vi "HEWH Get Statistics.vi"(4 "Flow Selector":T1, 6 "Emerson Flow Meter Data Output":T2, 8 "Error In":errorcluster, 10 "Elapsed Time (sec)":dbl, 11 "Core HEWH Data in":T3 {"Test Patten Setup"."PRAT/RLT Sequence"."Time" format="%<%H:%M:%S>t"; "Test Patten Setup"."Total Gallons Schedule" format="%.2f"}) -> (0 "Error Out":errorcluster, 1 "Mean,SD,Var,Max,Min Array":string[][](array[string]), 3 "Draw Stats Out":dbl[][](array[numeric]))   [LabVIEW 2016]
uses:
  Type Definitions/HEWH Output Information.ctl
  Type Definitions/HEWH Draw Pattern Setup.ctl
  Type Definitions/PRAT Test.ctl
  Utility/Save File/File Setup (Public)/Type Definition/Save File HEWH Heating Control Mode.ctl
  Draw Water Specific/Type Definitions/Terminate Draw Conditions.ctl
  Type Definitions/HEWH Start Conditions.ctl
  Draw Water Specific/Type Definitions/Check Special Condtions.ctl
  Draw Water Specific/Type Definitions/HEWH Special Condition Check.ctl
  Type Definitions/HEWH Draw Flag ENUM.ctl
  Type Definitions/HEWH Specific DAQ.ctl
  Type Definitions/HEWH Power Data.ctl
  Type Definitions/HEWH Power Elements.ctl
  Utility/Type Definitions/UTILITY Power Analyzer.ctl
  Type Definitions/HEWH Calc and Calibration.ctl
  Utility/Save File/File Setup (Public)/Type Definition/Save File DOE LabView Program.ctl
  Custom Instrument Control/MW100/Type Definitions/Station ID Selector.ctl
  Range/Type Definitions/RANGE ANSI Rate.ctl
  Drivers/Emerson 5700 Transmitter/Type Definitions/Emerson 5700 Data.ctl
  Type Definitions/Flow Meter Selector.ctl
  Utility/Save File/File Setup.lvlib
panel:
  # "Draw Pattern Setup (24 Hour)"
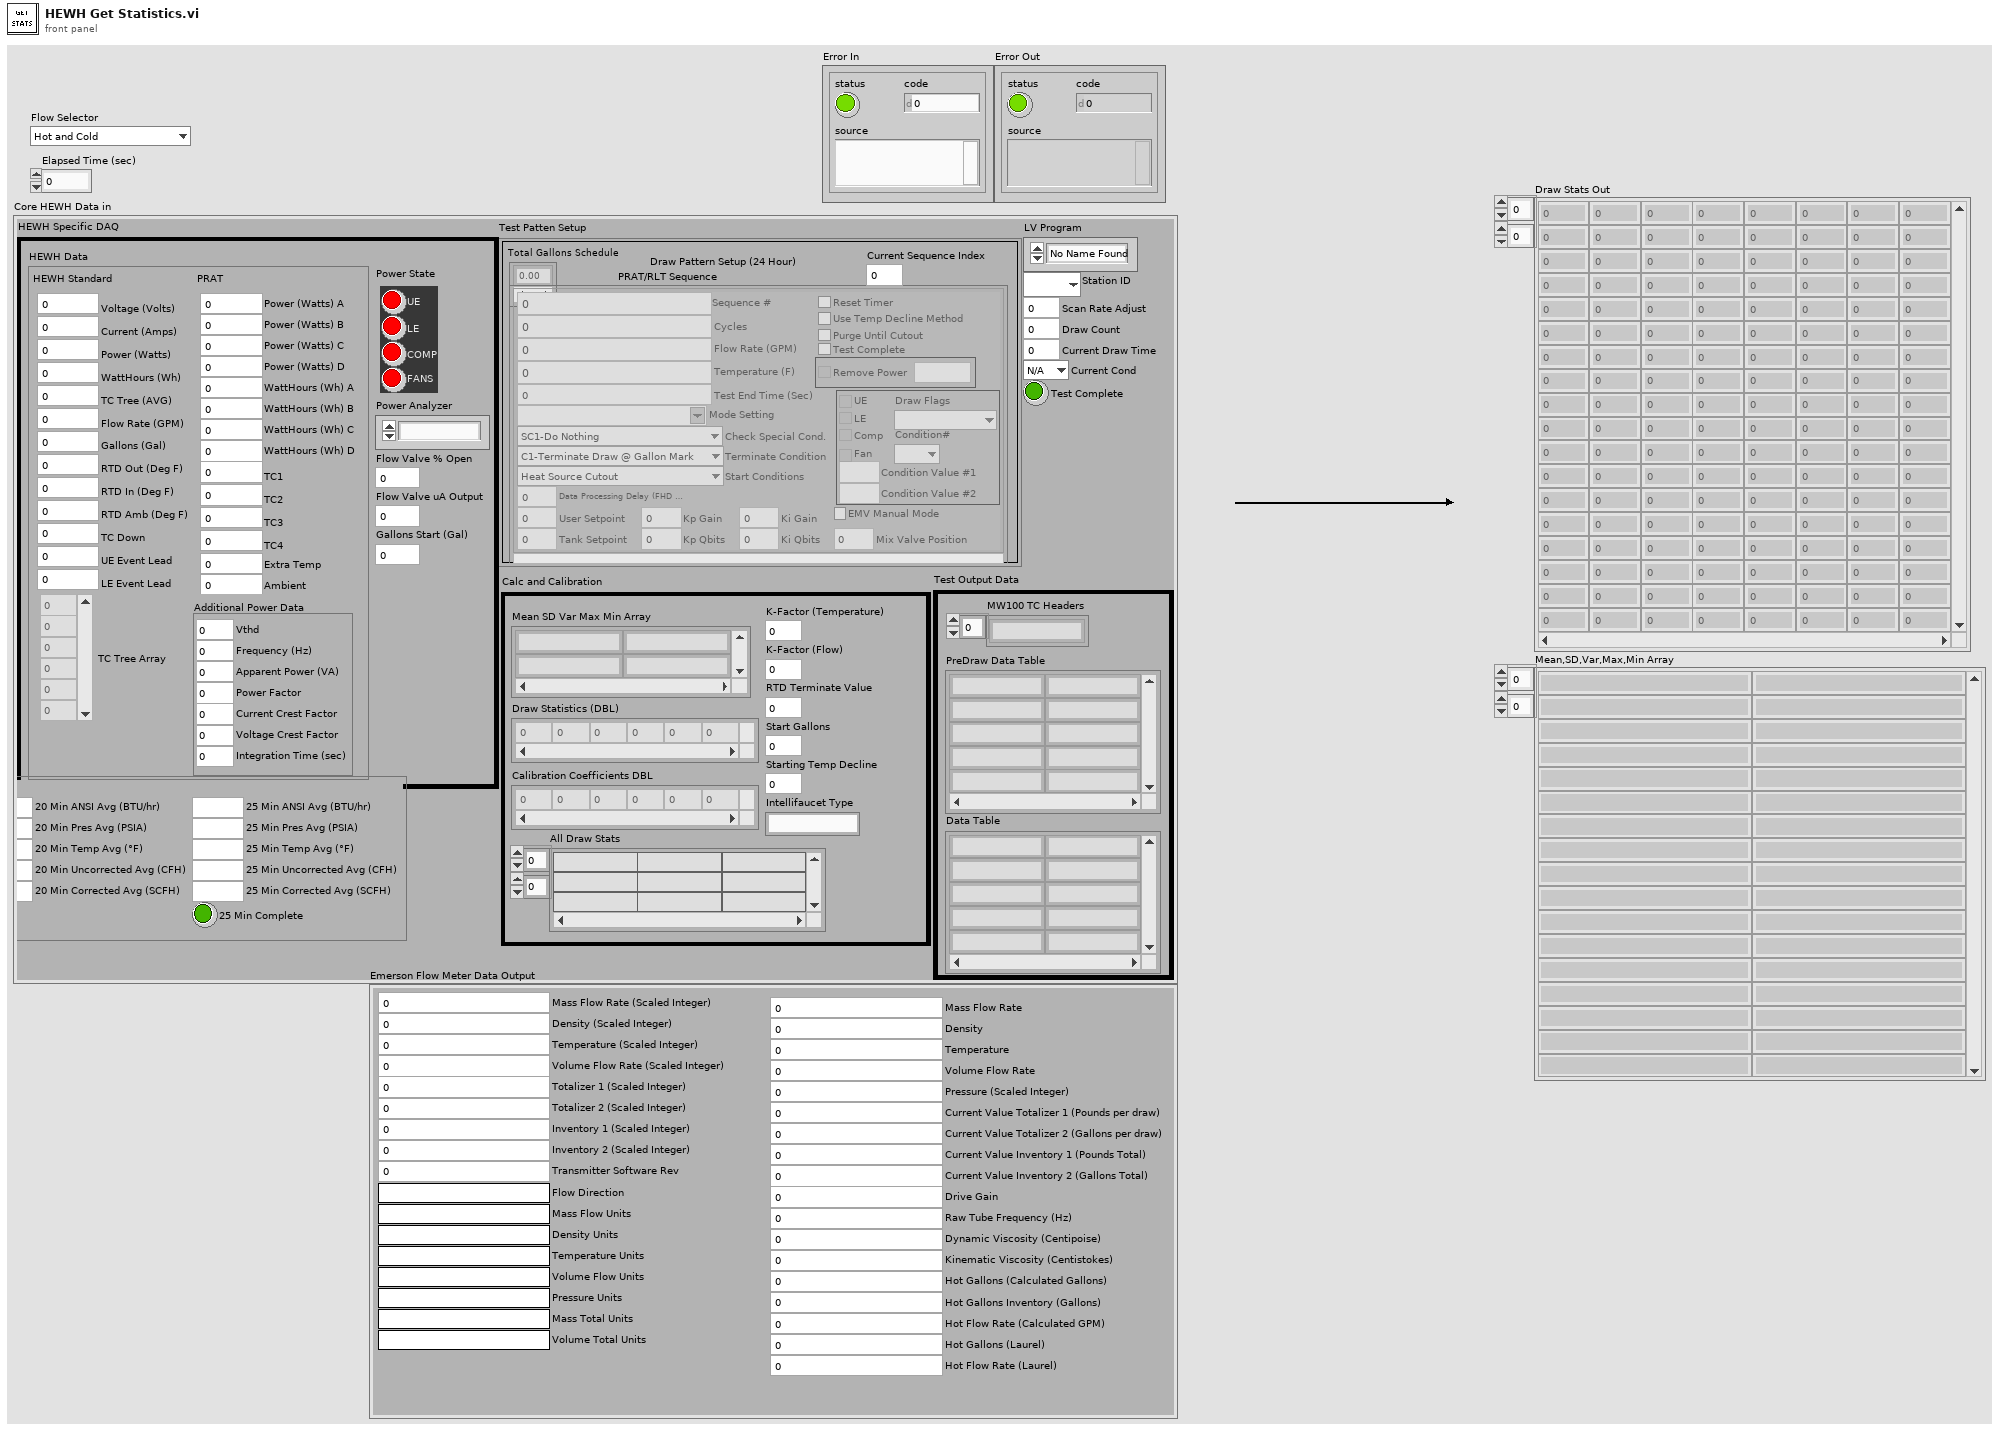
[diagram p1: front panel]
types:
  T1 = typedef "Flow Meter Selector.ctl" = enum16{"Hot and Cold", "Hot", "Cold", "None"}
  T2 = typedef "Emerson 5700 Data.ctl" = cluster{"Mass Flow Rate (Scaled Integer)":u16, "Density (Scaled Integer)":u16, "Temperature (Scaled Integer)":u16, "Volume Flow Rate (Scaled Integer)":u16, "Totalizer 1 (Scaled Integer)":u16, "Totalizer 2 (Scaled Integer)":u16, "Transmitter Software Rev":u16, "Flow Direction":string, "Mass Flow Units":string, "Density Units":string, "Temperature Units":string, "Volume Flow Units":string, "Pressure Units":string, "Mass Total Units":string, "Volume Total Units":string, "Inventory 1 (Scaled Integer)":u16, "Inventory 2 (Scaled Integer)":u16, "Mass Flow Rate":dbl, "Density":dbl, "Temperature":dbl, "Volume Flow Rate":dbl, "Pressure (Scaled Integer)":u16, "Current Value Totalizer 1 (Pounds per draw)":dbl, "Current Value Totalizer 2 (Gallons per draw)":dbl, "Current Value Inventory 1 (Pounds Total)":dbl, "Current Value Inventory 2 (Gallons Total)":dbl, "Drive Gain":dbl, "Raw Tube Frequency (Hz)":dbl, "Dynamic Viscosity (Centipoise)":dbl, "Kinematic Viscosity (Centistokes)":dbl, "Hot Gallons (Calculated Gallons)":dbl, "Hot Flow Rate (Calculated GPM)":dbl, "Hot Gallons Inventory (Gallons)":dbl, "Hot Flow Rate (Laurel)":dbl, "Hot Gallons (Laurel)":dbl}
  T3 = typedef "HEWH Output Information.ctl" = cluster{"Scan Rate Adjust":dbl, "Draw Count":i32, "Test Patten Setup":T4, "HEWH Specific DAQ":T12, "Test Output Data":cluster{"PreDraw Data Table":string[][], "Data Table":string[][], "MW100 TC Headers":string[]}, "Calc and Calibration":T16, "Current Draw Time":dbl, "LV Program":T17, "Station ID":T18, "Current Cond":T10, "Test Complete":bool, "ANSI Rate":T19}
  T4 = typedef "HEWH Draw Pattern Setup.ctl" = cluster{"Total Gallons Schedule":dbl[], "PRAT/RLT Sequence":T5[], "Current Sequence Index":i32}
  T5 = typedef "PRAT Test.ctl" = cluster{"Sequence #":dbl, "Cycles":i32, "Mode Setting":T6, "Flow Rate (GPM)":dbl, "Temperature (F)":dbl, "Reset Timer":bool, "Use Temp Decline Method":bool, "Terminate Condition":T7, "Condition Value #1":dbl, "UE":bool, "LE":bool, "Comp":bool, "Fan":bool, "Test End Time (Sec)":dbl, "Purge Until Cutout":bool, "Start Conditions":T8, "Condition Value #2":dbl, "Remove Power":bool, "Time":dbl, "Check Special Cond.":T9, "Condition#":T10, "Draw Flags":T11, "Data Processing Delay (FHD 15sec, UEF 5 Sec)":dbl, "Test Complete":bool, "User Setpoint":dbl, "Tank Setpoint":dbl, "Kp Gain":dbl, "Kp Qbits":dbl, "Ki Gain":dbl, "Ki Qbits":dbl, "Mix Valve Position":i16, "EMV Manual Mode":bool}
  T6 = typedef "File Setup.lvlib/Save File HEWH Heating Control Mode.ctl" = string
  T7 = typedef "Terminate Draw Conditions.ctl" = enum16{"C1-Terminate Draw @ Gallon Mark", "C2-Special Last Draw (HU Test)", "C3-RTD Out <=", "C4-Mean Tank Temp <=", "C5-Decrease RTD Out (Deg F)", "C6-Time (Seconds)", "C7-Until Any Heat Source", "C8-Specific Heat Source", "C9-Do Nothing"}
  T8 = typedef "HEWH Start Conditions.ctl" = enum16{"Heat Source Cutout", "At Time (Seconds)", "Every X (Seconds)", "T2 >= X° Below Setpoint", "Seconds From Complete", "Wait for LE & Comp Cutout", "Wait for Comp Cutout", "Wait for LE Cutout", "Wait for UE Cutout"}
  T9 = typedef "Check Special Condtions.ctl" = enum16{"SC1-Do Nothing", "SC2-Check Heat Source (On-C2/Off-C1)", "SC3-Check Skip Condition", "SC4-Check Heat Source ON/Fail"}
  T10 = typedef "HEWH Special Condition Check.ctl" = enum16{"N/A", "C1", "C2", "Reset/Fail", "Skip Draw Sequence"}
  T11 = typedef "HEWH Draw Flag ENUM.ctl" = enum16{"N/A", "None(0)", "Sml(1)", "Med(2)", "SmlMed(3)", "Lrg(4)", "SmlLrg(5)", "MedLrg(6)", "SmlMedLrg(7)"}
  T12 = typedef "HEWH Specific DAQ.ctl" = cluster{"HEWH Data":T13, "Flow Valve % Open":dbl, "Power State":T14, "Power Analyzer":T15, "Flow Valve uA Output":i32, "Gallons Start (Gal)":dbl}
  T13 = typedef "HEWH Power Data.ctl" = cluster{"HEWH Standard":cluster{"Voltage (Volts)":dbl, "Current (Amps)":dbl, "Power (Watts)":dbl, "WattHours (Wh)":dbl, "TC Tree (AVG)":dbl, "Flow Rate (GPM)":dbl, "Gallons (Gal)":dbl, "RTD Out (Deg F)":dbl, "RTD In (Deg F)":dbl, "RTD Amb (Deg F)":dbl, "TC Down":dbl, "UE Event Lead":i32, "LE Event Lead":i32, "TC Tree Array":dbl[]}, "PRAT":cluster{"Power (Watts) A":dbl, "Power (Watts) B":dbl, "Power (Watts) C":dbl, "Power (Watts) D":dbl, "TC1":dbl, "TC2":dbl, "TC3":dbl, "TC4":dbl, "WattHours (Wh) A":dbl, "WattHours (Wh) B":dbl, "WattHours (Wh) C":dbl, "WattHours (Wh) D":dbl, "Ambient":dbl, "Extra Temp":dbl}, "Additional Power Data":cluster{"Vthd":dbl, "Frequency (Hz)":dbl, "Apparent Power (VA)":dbl, "Power Factor":dbl, "Current Crest Factor":dbl, "Voltage Crest Factor":dbl, "Integration Time (sec)":dbl}}
  T14 = typedef "HEWH Power Elements.ctl" = cluster{"UE":bool, "LE":bool, "COMP":bool, "FANS":bool}
  T15 = typedef "UTILITY Power Analyzer.ctl" = enum16{"", "APLUS", "WT210", "WT500", "WT300", "OSI", "Debug", "WT230", "WT300_1", "WT300_2"}
  T16 = typedef "HEWH Calc and Calibration.ctl" = cluster{"Mean SD Var Max Min Array":string[][], "Draw Statistics (DBL)":dbl[][], "Calibration Coefficients DBL":dbl[][], "Start Gallons":dbl, "Starting Temp Decline":dbl, "K-Factor (Temperature)":dbl, "All Draw Stats":string[][], "RTD Terminate Value":dbl, "K-Factor (Flow)":dbl, "Intellifaucet Type":string}
  T17 = typedef "File Setup.lvlib/Save File DOE LabView Program.ctl" = enum16{"No Name Found", "DOE Stand", "Dishwasher Kitchen", "Portable Stand", "HEWH", "Dryer", "Dryer WILT", "HCC", "PRAT", "HEWH RLT", "Refrigeration"}
  T18 = typedef "Station ID Selector.ctl" = enum16{"", "A", "B", "C", "D", "Global"}
  T19 = typedef "RANGE ANSI Rate.ctl" = cluster{"Array 1":dbl[], "Array 3":dbl[], "Array 2":dbl[], "Start ANSI":bool, "ANSI Start Time":dbl, "Restart ANSI":bool, "15 Min ANSI Avg (BTU/hr)":dbl, "20 Min ANSI Avg (BTU/hr)":dbl, "25 Min ANSI Avg (BTU/hr)":dbl, "Absolute Pressure":dbl, "Gas Temperature":dbl, "Volumetric Flow Rate":dbl, "Mass Flow Rate":dbl, "Array 4":dbl[], "Array 5":dbl[], "Gas Rate":dbl, "15 Min Pres Avg (PSIA)":dbl, "20 Min Pres Avg (PSIA)":dbl, "25 Min Pres Avg (PSIA)":dbl, "15 Min Temp Avg (°F) ":dbl, "20 Min Temp Avg (°F)":dbl, "25 Min Temp Avg (°F)":dbl, "15 Min Uncorrected Avg (CFH)":dbl, "20 Min Uncorrected Avg (CFH)":dbl, "25 Min Uncorrected Avg (CFH)":dbl, "15 Min Corrected Avg (SCFH)":dbl, "20 Min Corrected Avg (SCFH)":dbl, "25 Min Corrected Avg (SCFH)":dbl, "15 Min Complete":bool, "20 Min Complete":bool, "25 Min Complete":bool}
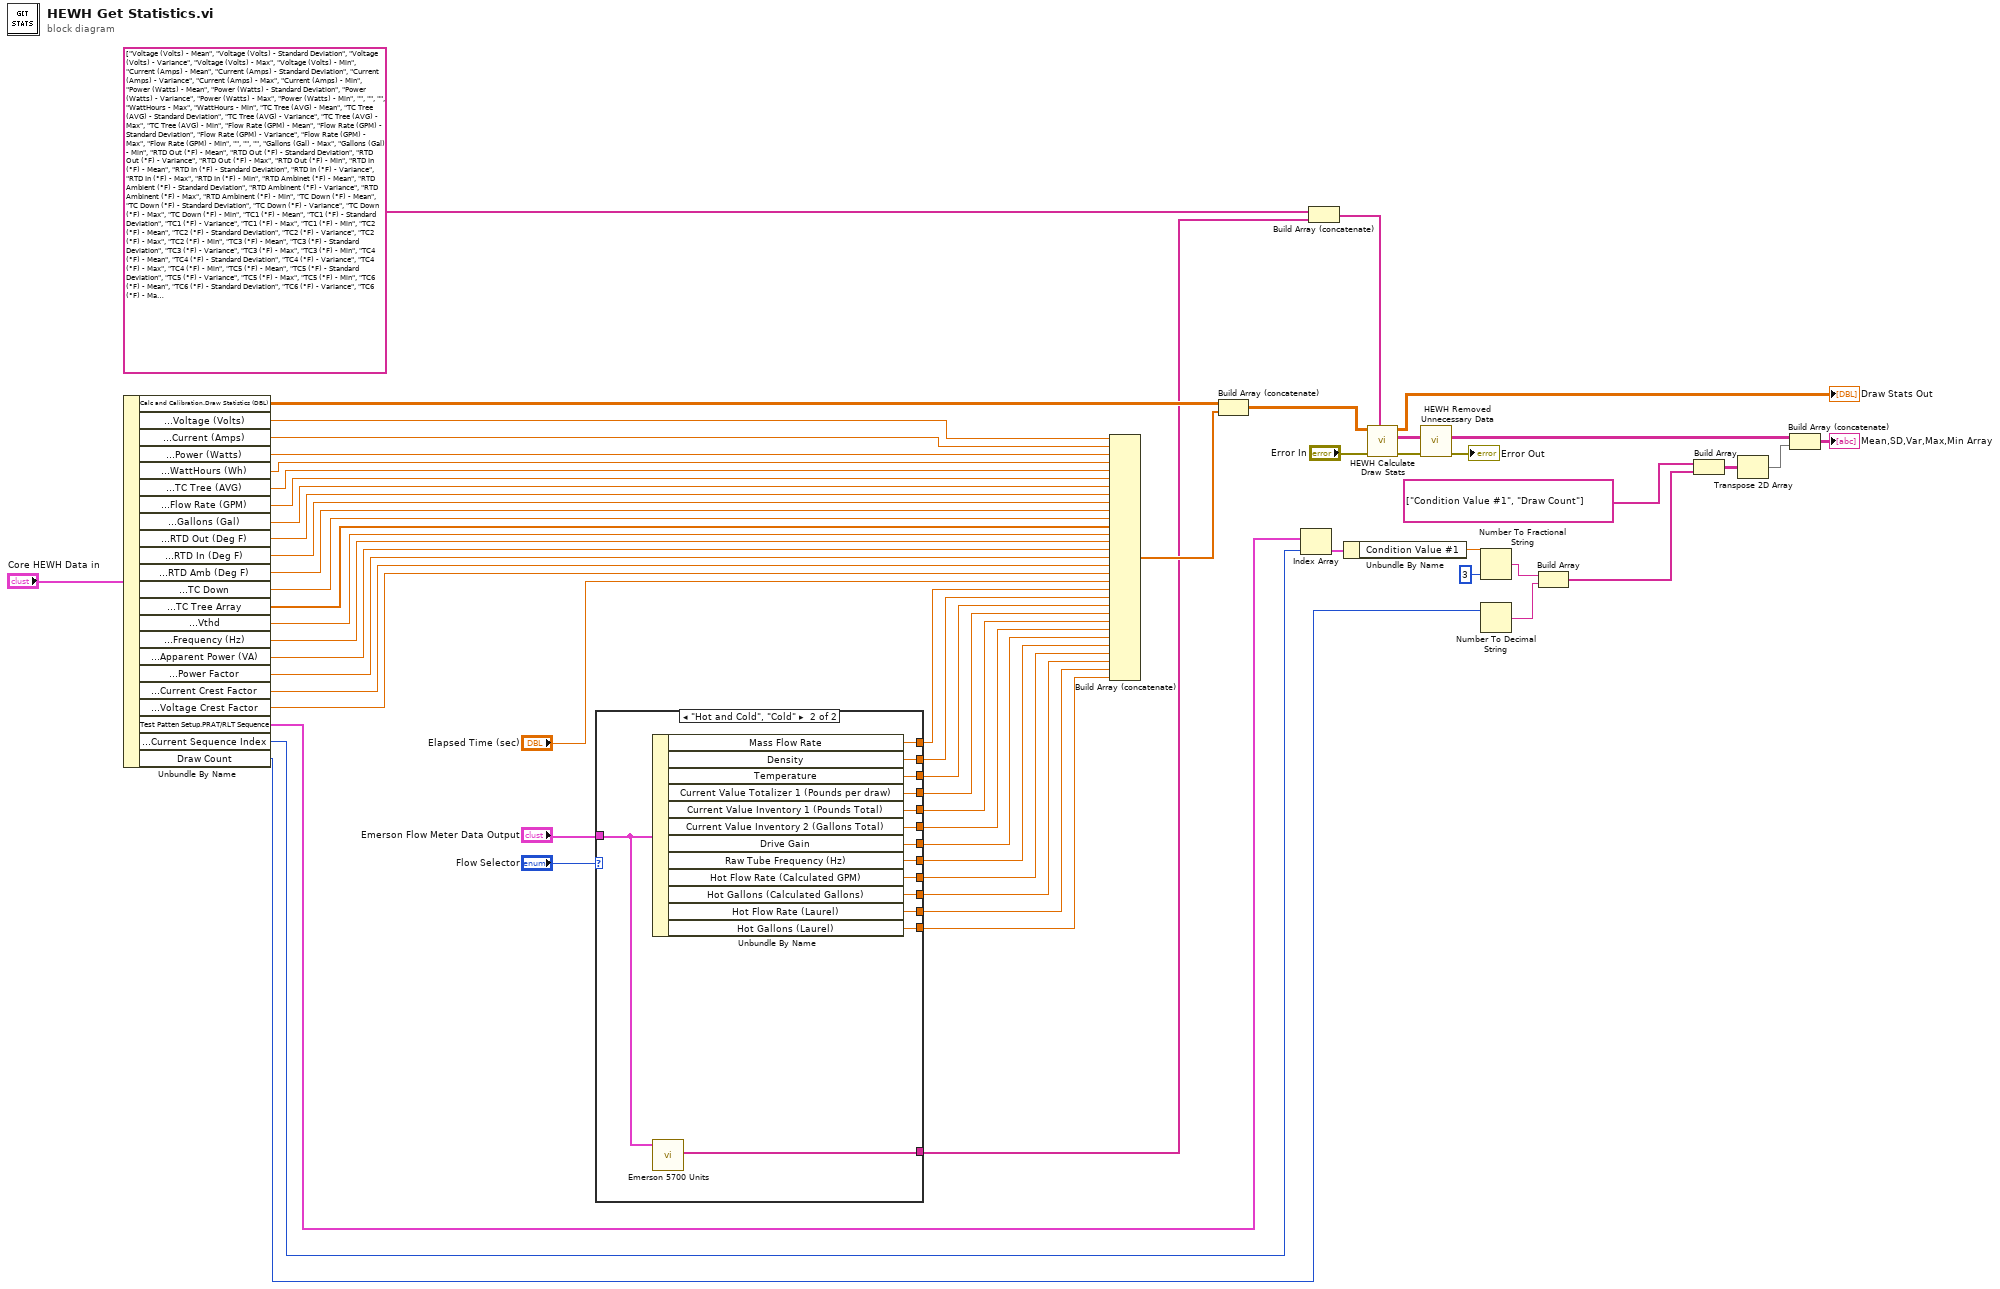
[diagram p0: block diagram]
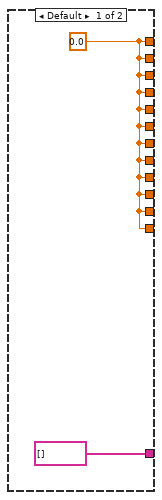
[diagram p2: hidden frame]
diagram:
  n1 = Unbundle By Name("Core HEWH Data in") -> ("Calc and Calibration.Draw Statistics (DBL)"=w50:dbl[][], "HEWH Specific DAQ.HEWH Data.HEWH Standard.Voltage (Volts)"=w31:dbl, "HEWH Specific DAQ.HEWH Data.HEWH Standard.Current (Amps)"=w32:dbl, "HEWH Specific DAQ.HEWH Data.HEWH Standard.Power (Watts)"=w33:dbl, "HEWH Specific DAQ.HEWH Data.HEWH Standard.WattHours (Wh)"=w34:dbl, "HEWH Specific DAQ.HEWH Data.HEWH Standard.TC Tree (AVG)"=w35:dbl, "HEWH Specific DAQ.HEWH Data.HEWH Standard.Flow Rate (GPM)"=w36:dbl, "HEWH Specific DAQ.HEWH Data.HEWH Standard.Gallons (Gal)"=w37:dbl, "HEWH Specific DAQ.HEWH Data.HEWH Standard.RTD Out (Deg F)"=w38:dbl, "HEWH Specific DAQ.HEWH Data.HEWH Standard.RTD In (Deg F)"=w39:dbl, "HEWH Specific DAQ.HEWH Data.HEWH Standard.RTD Amb (Deg F)"=w40:dbl, "HEWH Specific DAQ.HEWH Data.HEWH Standard.TC Down"=w41:dbl, "HEWH Specific DAQ.HEWH Data.HEWH Standard.TC Tree Array"=w42:dbl[], "HEWH Specific DAQ.HEWH Data.Additional Power Data.Vthd"=w43:dbl, "HEWH Specific DAQ.HEWH Data.Additional Power Data.Frequency (Hz)"=w44:dbl, "HEWH Specific DAQ.HEWH Data.Additional Power Data.Apparent Power (VA)"=w45:dbl, "HEWH Specific DAQ.HEWH Data.Additional Power Data.Power Factor"=w46:dbl, "HEWH Specific DAQ.HEWH Data.Additional Power Data.Current Crest Factor"=w47:dbl, "HEWH Specific DAQ.HEWH Data.Additional Power Data.Voltage Crest Factor"=w48:dbl, "Test Patten Setup.PRAT/RLT Sequence"=w52:T5[], "Test Patten Setup.Current Sequence Index"=w53:i32, "Draw Count"=w25:i32)
  n2 = case shown="\"Hot and Cold\", \"Cold\"" "Flow Selector" {
    tunnel: "Emerson Flow Meter Data Output" -> [_ w75]
    tunnel: [string[] [] w74] -> w8
    tunnel: [w60 w73] -> w16
    tunnel: [w60 w72] -> w15
    tunnel: [w60 w71] -> w14
    tunnel: [w60 w70] -> w13
    tunnel: [w60 w69] -> w12
    tunnel: [w60 w68] -> w11
    tunnel: [w60 w67] -> w7
    tunnel: [w60 w66] -> w6
    tunnel: [w60 w65] -> w5
    tunnel: [w60 w64] -> w4
    tunnel: [w60 w63] -> w3
    tunnel: [w60 w62] -> w1
    frame Default {
      w60 = 0.0 ("Mass Flow Rate")
    }
    frame "Hot and Cold", "Cold" {
      n3 = Unbundle By Name(w75) -> ("Mass Flow Rate"=w73:dbl, "Density"=w72:dbl, "Temperature"=w71:dbl, "Current Value Totalizer 1 (Pounds per draw)"=w70:dbl, "Current Value Inventory 1 (Pounds Total)"=w69:dbl, "Current Value Inventory 2 (Gallons Total)"=w68:dbl, "Drive Gain"=w67:dbl, "Raw Tube Frequency (Hz)"=w66:dbl, "Hot Flow Rate (Calculated GPM)"=w65:dbl, "Hot Gallons (Calculated Gallons)"=w64:dbl, "Hot Flow Rate (Laurel)"=w63:dbl, "Hot Gallons (Laurel)"=w62:dbl)
      n4 = call "Emerson 5700 Units.vi"("Emerson Flow Meter Data Input"=w75) -> ("Units with Mean, STD, ect"=w74:string[])  [unwired: 7 in, 3 out]
    }
  }
  n5 = Build Array (concatenate)(w31, w32, w33, w34, w35, w36, w37, w38, w39, w40, w41, w42, w43, w44, w45, w46, w47, w48, "Elapsed Time (sec)", w16, w15, w14, w13, w12, w11, w7, w6, w5, w4, w3, w1) -> (w49:dbl[])
  n6 = Build Array (concatenate)(w50, w49) -> (w59:dbl[][])
  n7 = Index Array(array=w52, index=w53) -> (element=w51:T5)
  n8 = Build Array (concatenate)(string[] ["Voltage (Volts) - Mean", "Voltage (Volts) - Standard Deviation", "Voltage (Volts) - Variance", "Voltage (Volts) - Max", "Voltage (Volts) - Min", "Current (Amps) - Mean", "Current (Amps) - Standard Deviation", "Current (Amps) - Variance", "Current (Amps) - Max", "Current (Amps) - Min", "Power (Watts) - Mean", "Power (Watts) - Standard Deviation", "Power (Watts) - Variance", "Power (Watts) - Max", "Power (Watts) - Min", "", "", "", "WattHours - Max", "WattHours - Min", "TC Tree (AVG) - Mean", "TC Tree (AVG) - Standard Deviation", "TC Tree (AVG) - Variance", "TC Tree (AVG) - Max", "TC Tree (AVG) - Min", "Flow Rate (GPM) - Mean", "Flow Rate (GPM) - Standard Deviation", "Flow Rate (GPM) - Variance", "Flow Rate (GPM) - Max", "Flow Rate (GPM) - Min", "", "", "", "Gallons (Gal) - Max", "Gallons (Gal) - Min", "RTD Out (°F) - Mean", "RTD Out (°F) - Standard Deviation", "RTD Out (°F) - Variance", "RTD Out (°F) - Max", "RTD Out (°F) - Min", "RTD In (°F) - Mean", "RTD In (°F) - Standard Deviation", "RTD In (°F) - Variance", "RTD In (°F) - Max", "RTD In (°F) - Min", "RTD Ambinet (°F) - Mean", "RTD Ambient (°F) - Standard Deviation", "RTD Ambinent (°F) - Variance", "RTD Ambinent (°F) - Max", "RTD Ambinent (°F) - Min", "TC Down (°F) - Mean", "TC Down (°F) - Standard Deviation", "TC Down (°F) - Variance", "TC Down (°F) - Max", "TC Down (°F) - Min", "TC1 (°F) - Mean", "TC1 (°F) - Standard Deviation", "TC1 (°F) - Variance", "TC1 (°F) - Max", "TC1 (°F) - Min", "TC2 (°F) - Mean", "TC2 (°F) - Standard Deviation", "TC2 (°F) - Variance", "TC2 (°F) - Max", "TC2 (°F) - Min", "TC3 (°F) - Mean", "TC3 (°F) - Standard Deviation", "TC3 (°F) - Variance", "TC3 (°F) - Max", "TC3 (°F) - Min", "TC4 (°F) - Mean", "TC4 (°F) - Standard Deviation", "TC4 (°F) - Variance", "TC4 (°F) - Max", "TC4 (°F) - Min", "TC5 (°F) - Mean", "TC5 (°F) - Standard Deviation", "TC5 (°F) - Variance", "TC5 (°F) - Max", "TC5 (°F) - Min", "TC6 (°F) - Mean", "TC6 (°F) - Standard Deviation", "TC6 (°F) - Variance", "TC6 (°F) - Max", "TC6 (°F) - Min", "", "", "", "Total Harmonic Distortion (%V) - Max", "Total Harmonic Distortion (%V) - Min", "Frequency (Hz) - Mean ", "Frequency (Hz) - Standard Deviation", "Frequency (Hz) - Variance", "Frequency (Hz) - Max", "Frequency (Hz) - Min", "Apparent Power (VA) - Mean", "Apparent Power (VA) - Standard Deviation", "Apparent Power (VA) - Variance", "Apparent Power (VA) - Max", "Apparent Power (VA) - Min", "", "", "", "Power Factor - Max", "Power Factor - Min", "", "", "", "Current Crest Factor - Max", "Current Crest Factor - Min", "", "", "", "Voltage Crest Factor - Max", "Voltage Crest Factor - Min", "", "", "", "Elapsed Time (Sec) - Max", "Elapsed Time (Sec) - Min"], w8) -> (w9:string[])
  n9 = Unbundle By Name(w51) -> ("Condition Value #1"=w27:dbl)
  n10 = call "HEWH Calculate Draw Stats.vi"("Headers"=w9, "Error In"="Error In", "Draw Stats"=w59) -> ("Error Out"=w58:errorcluster, "Data With Headers"=w55:string[][], "Draw Stats Out"=→"Draw Stats Out":dbl[][])  [unwired: 6 in]
  n11 = call "HEWH Removed Unnecessary Data.vi"("Error In"=w58, "Data With Headers"=w55) -> ("Error Out"=→"Error Out":errorcluster, "Stat Data Output"=w22:string[][])  [unwired: 7 in, 1 out]
  n12 = Number To Fractional String(number=w27, precision (6)=i16 3) -> (F-format string=w26:string)  [unwired: 2 in]
  n13 = Number To Decimal String(number=w25) -> (decimal integer string=w24:string)  [unwired: 1 in]
  n14 = Build Array(w26, w24) -> (w23:string[])
  n15 = Build Array(string[] ["Condition Value #1", "Draw Count"], w23) -> (w20:string[][])
  n16 = Transpose 2D Array(2D array=w20) -> (transposed array=w19:string[][])
  n17 = Build Array (concatenate)(w22, w19) -> (→"Mean,SD,Var,Max,Min Array":string[][])
